vi "audio-stim2.vi"(11 "Stimulus List":dbl[][](array[numeric])=[[1.0, 3.0, 0.2, 1.0, 50.0], [2.0, 3.0, 0.2, 1.0, 100.0], [3.0, 3.0, 0.2, 1.0, 200.0], [4.0, 3.0, 0.2, 1.0, 400.0], [5.0, 3.0, 0.2, 1.0, 800.0], [6.0, 3.0, 0.2, 1.0, 1600.0], [7.0, 3.0, 0.2, 1.0, 3200.0], [8.0, 3.0, 0.2, 1.0, 6400.0], [9.0, 3.0, 0.2, 1.0, 9050.9668], [10.0, 3.0, 0.2, 1.0, 128000.0], [11.0, 3.0, 0.2, 1.0, 18101.9336], [12.0, 3.0, 0.2, 1.0, 256000.0], [13.0, 3.0, 0.2, 1.0, 36203.8672]]) -> (3 "Playing":bool=TRUE caption="Playing stimulus")   [LabVIEW 2013]
uses:
  <vilib>/DAQmx/write.llb/DAQmx Write (Digital U16 1Chan 1Samp).vi
  <vilib>/DAQmx/write.llb/DAQmx Write (Analog Wfm 1Chan NSamp).vi
  <vilib>/DAQmx/create/channels.llb/DAQmx Create Channel (AO-Voltage-Basic).vi
  <vilib>/DAQmx/create/channels.llb/DAQmx Create Channel (DO-Digital Output).vi
  <vilib>/DAQmx/miscellaneous.llb/DAQmx Fill In Error Info.vi
  <vilib>/DAQmx/configure/timing.llb/DAQmx Timing (Use Waveform).vi
panel:
  in  "Total Trials":i32=2147483647 min=1 step=1
  out "Total Played":i32 caption="Total Played or Cued"
  in  "Save Stimulus List":bool
  in  "Load Stimulus List":bool
  out "Stimulus List Path":path
  out "Log File Path":path
  in  "Play Interval Jitter (s)":dbl=0.5
  in  "Play Interval (s)":dbl=1.0
  out "error out":errorcluster
  in  "DO Ports":tag="Dev1/port0" caption="DO Ports\n(\"browse\" and select two 8 bit ports)"
  in  "Sound AO Channel":tag="Dev1/ao0"
  out "Curr Param":dbl[](array[numeric]) caption="Current (or Cued) Trial Parameters"
  in  "Sampling Rate":dbl=100000.0
  in  "stop":bool
  in  "Play":bool
  out "Current (or Cued) Waveform":waveform(dbl)(graph)={"t0"=timestamp(0 s since 1904-01-01), "dt"=1e-05, "Y"=array[19999 elements]}
  out "Waiting":bool=TRUE
  # "Stim#, Stim Type, Duration, Amplitude, Param 1, Param 2, Param 3, Param 4"
  # "Stim Type 1 DC (no parameters, just amplitude)"
  # "Stim Type 3 Pure Tone (param1 = frequency)"
  # "Stim Type 4 FM Sweep (param1 = start frequency, param2 = end frequency)"
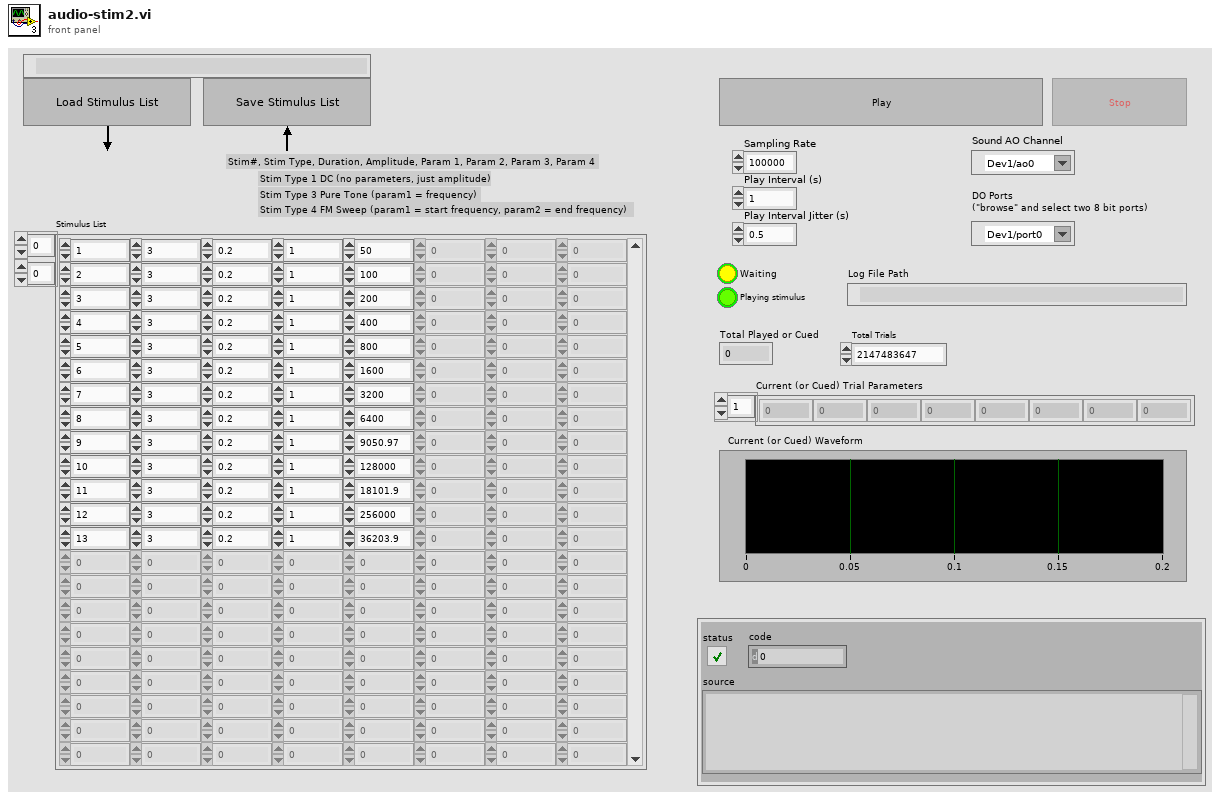
[diagram p1: front panel]
types:
  T1 = enum8{"Enabled", "Disabled", "Disabled and Grayed Out"}
  T2 = cluster{"Sampling Rate":dbl, "Value 3":dbl, dbl, "Value 2":dbl}
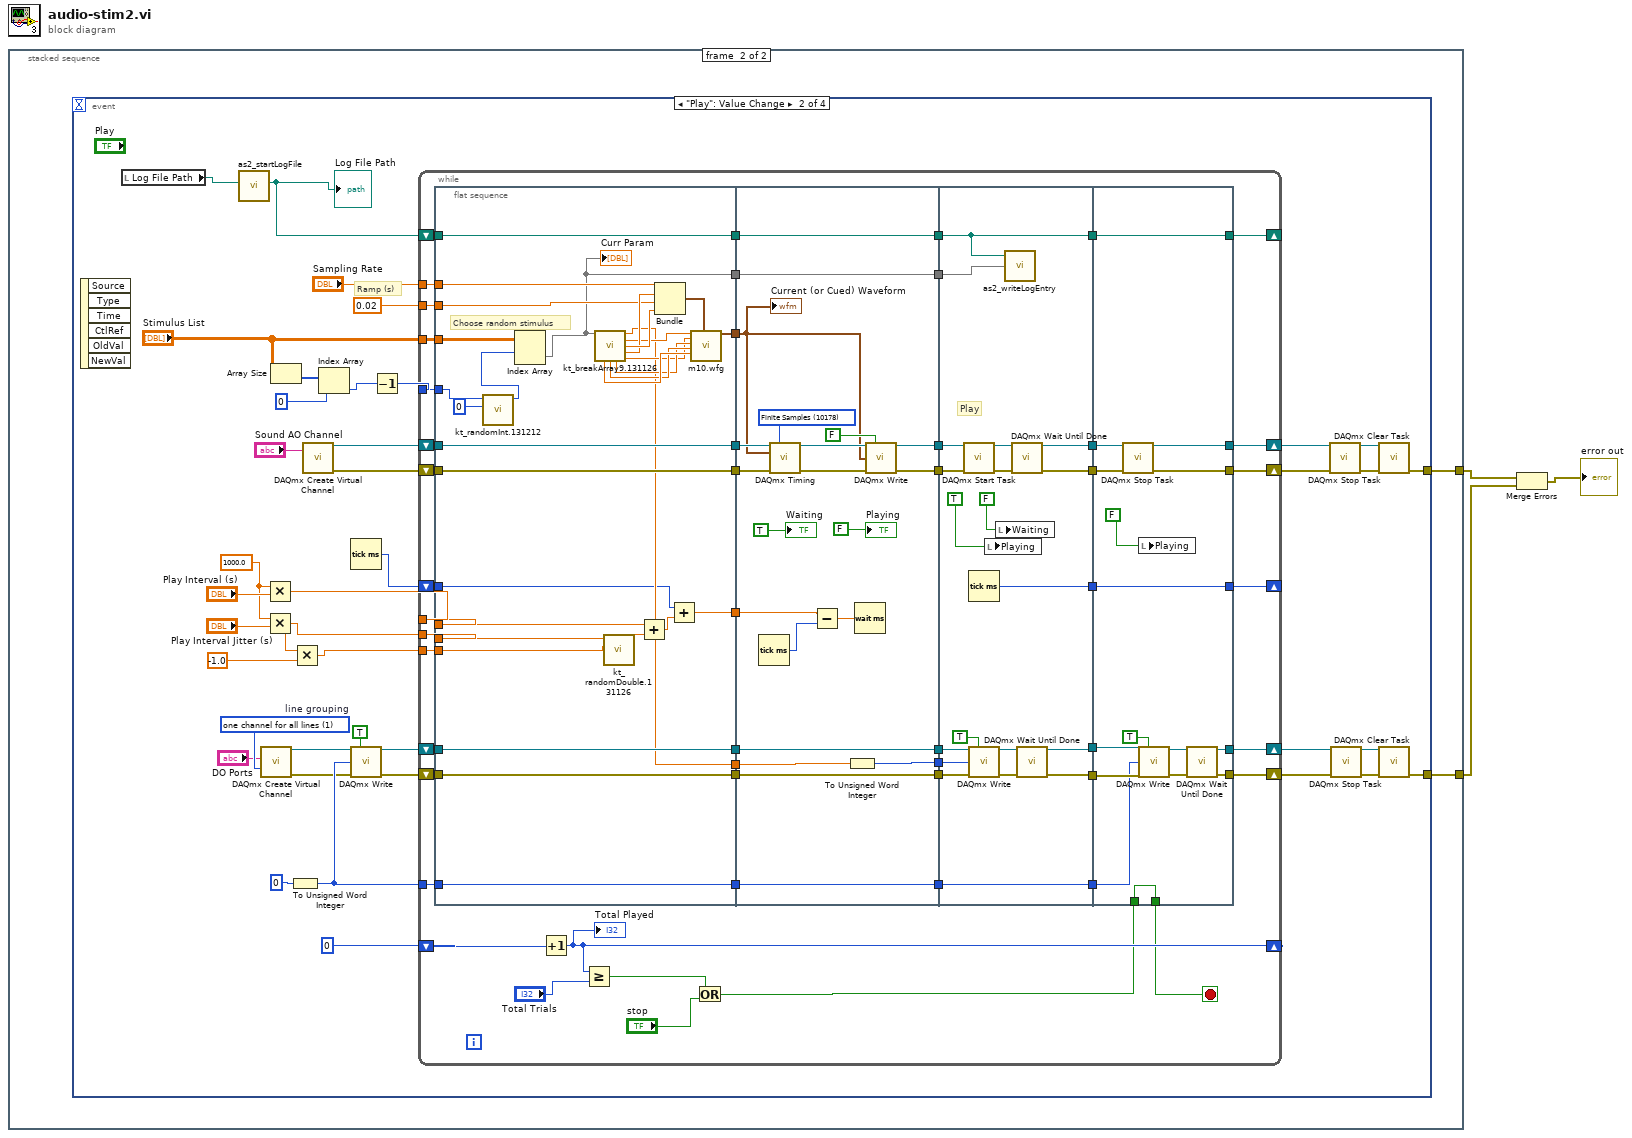
[diagram p0: block diagram]
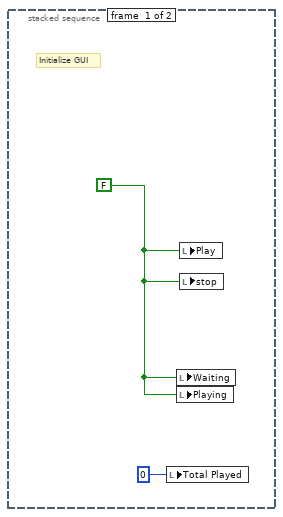
[diagram p2: hidden frame]
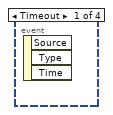
[diagram p3: hidden frame]
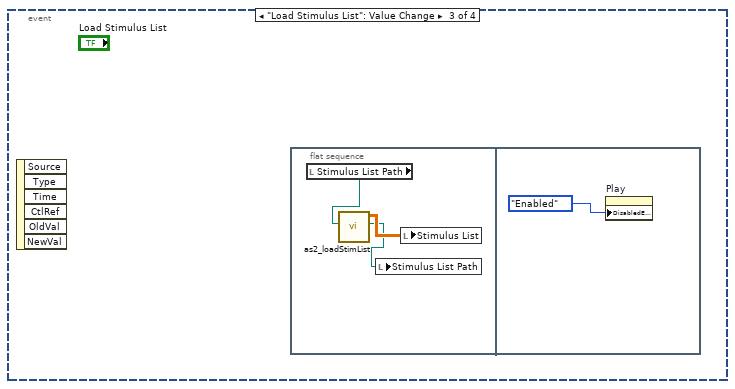
[diagram p4: hidden frame]
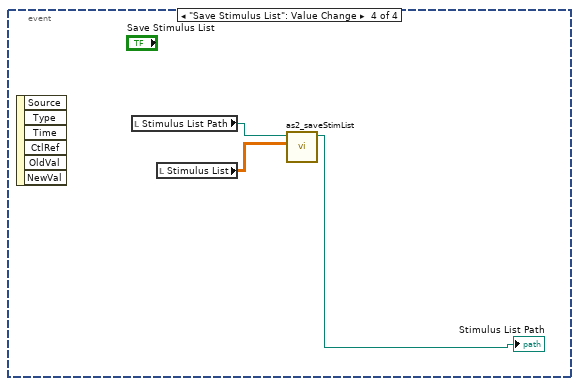
[diagram p5: hidden frame]
diagram:
  n1 = stacked-sequence {
    tunnel: [_ w7] -> w3
    tunnel: [_ w6] -> w2
    frame #0 {
      w5 = FALSE ("Play")
      # "Initialize GUI"
      n2 = local write "Total Played"(0 ("Total Played")) -> ()
      n3 = local write "Waiting"(w5) -> ()
      n4 = local write "Playing"(w5) -> ()
      n5 = local write "Play"(w5) -> ()
      n6 = local write "stop"(w5) -> ()
    }
    frame #1 {
      n7 = event shown="[1] \"Play\": Value Change" {
        selector: _ -> [_ _ _ _]
        dyn-events: _ -> [_ _ _ _]
        timeout: _ -> [_ _ _ _]
        tunnel: [_ w24 _ _] -> w7
        tunnel: [_ w23 _ _] -> w6
        event Timeout {
          n8 = event-data() -> ()  [unwired: 1 in, 3 out]
        }
        event "Play": Value Change {
          w17 = 1000.0 ("y")
          w44 = 1 items=["one channel for each line", "one channel for all lines"]  # line grouping
          # "Ramp (s)"
          n9 = event-data() -> ()  [unwired: 1 in, 6 out]
          n10 = local read "Log File Path"() -> (w12:path)
          n11 = call "as2_startLogFile.vi"("Path In"=w12) -> ("Path"=w11:path)  [unwired: 5 in, 1 out]
          "Log File Path" <- w11
          n12 = call-poly <vilib>:"DAQmx Create Virtual Channel.vi"("lines"="DO Ports", "line grouping"=w44) -> ("task out"=w22:refnum<k21>, "error out"=w21:errorcluster)  [unwired: 12 in]
          n13 = Multiply(x=w17, y="Play Interval (s)") -> (x*y=w16:dbl)
          n14 = Multiply(x=w17, y="Play Interval Jitter (s)") -> (x*y=w14:dbl)
          n15 = Array Size(array="Stimulus List") -> (size(s)=w42:i32[])
          n16 = To Unsigned Word Integer(number=u16 0 ("data")) -> (unsigned 16bit integer=w27:u16)
          n17 = Multiply(x=w14, y=-1.0) -> (x*y=w15:dbl)
          n18 = call-poly <vilib>:"DAQmx Create Virtual Channel.vi"("physical channels"="Sound AO Channel") -> ("task out"=w26:refnum<k21>, "error out"=w25:errorcluster)  [unwired: 13 in]
          n19 = Index Array(array=w42, index=0) -> (element=w10:i32)
          n20 = Tick Count (ms)() -> (millisecond timer value=w13:u32)
          n21 = call-poly <vilib>:"DAQmx Write.vi"("task/channels in"=w22, "auto start"=TRUE, "data"=w27, "error in"=w21) -> ("task out"=w31:refnum<k21>, "error out"=w30:errorcluster)  [unwired: 9 in, 1 out]
          n22 = Decrement(x=w10) -> (x-1=w9:i32)
          n23 = while {
            tunnel: "Stimulus List" -> [w72]
            tunnel: "Sampling Rate" -> [w71]
            tunnel: 0.02 -> [w70]
            shift-right: [w97] -> w36
            shift-left: w26 -> [w95]
            shift-right: [w96] -> w35
            shift-left: w25 -> [w94]
            shift-right: [w86] -> w40
            shift-left: w31 -> [w93]
            shift-right: [w85] -> w39
            shift-left: w30 -> [w80]
            shift-right: [w51] -> _
            shift-left: 0 ("data") -> [w52]
            tunnel: w27 -> [w83]
            shift-right: [w67] -> _
            shift-left: w13 -> [w66]
            tunnel: w16 -> [w62]
            tunnel: w15 -> [w63]
            tunnel: w14 -> [w64]
            shift-right: [w55] -> _
            shift-left: w11 -> [w61]
            tunnel: w9 -> [w54]
            stop <- w49 stop-if-true
            n24 = flat-sequence {
              tunnel: [w129] -> w78
              tunnel: [w128] -> w77
              tunnel: [w127] -> w76
              tunnel: [w126] -> w75
              tunnel: [w125] -> w74
              tunnel: [w117] -> w73
              tunnel: [w114] -> w69
              tunnel: [w111] -> w65
              tunnel: [w105] -> w60
              tunnel: [w104] -> w59
              tunnel: w54 -> [w103]
              tunnel: w61 -> [w105]
              tunnel: w62 -> [w106]
              tunnel: w63 -> [w109]
              tunnel: w64 -> [w110]
              tunnel: w66 -> [w112]
              tunnel: w70 -> [w115]
              tunnel: w71 -> [w116]
              tunnel: w72 -> [w101]
              tunnel: w80 -> [w125]
              tunnel: w83 -> [w126]
              tunnel: w93 -> [w127]
              tunnel: w94 -> [w128]
              tunnel: w95 -> [w129]
              tunnel: [w140] -> w99
              tunnel: [w139] -> w98
              tunnel: [w149] -> w92
              tunnel: [w148] -> w87
              tunnel: [w147] -> w84
              tunnel: [w137] -> w79
              tunnel: w78 -> [w146]
              tunnel: w77 -> [w145]
              tunnel: w76 -> [w149]
              tunnel: w75 -> [w147]
              tunnel: w74 -> [w137]
              tunnel: w73 -> [w136]
              tunnel: w69 -> [w135]
              tunnel: w65 -> [w132]
              tunnel: w60 -> [w130]
              tunnel: w59 -> [w131]
              tunnel: [w131] -> w58
              tunnel: [w130] -> w57
              tunnel: w99 -> [w160]
              tunnel: w98 -> [w159]
              tunnel: w92 -> [w168]
              tunnel: [w162] -> w91
              tunnel: [w161] -> w90
              tunnel: [w165] -> w89
              tunnel: [w164] -> w88
              tunnel: w87 -> [w169]
              tunnel: w84 -> [w163]
              tunnel: [w163] -> w82
              tunnel: w79 -> [w154]
              tunnel: [w153] -> w68
              tunnel: w58 -> [w152]
              tunnel: w57 -> [w151]
              tunnel: [w151] -> w56
              tunnel: [w174] -> w96
              tunnel: [w175] -> w97
              tunnel: w91 -> [w177]
              tunnel: w90 -> [w176]
              tunnel: w89 -> [w185]
              tunnel: w88 -> [w184]
              tunnel: [w180] -> w86
              tunnel: [w179] -> w85
              tunnel: w82 -> [w178]
              tunnel: w68 -> [w173]
              tunnel: [w173] -> w67
              tunnel: w56 -> [w172]
              tunnel: [w172] -> w55
              tunnel: w50 -> [w171]
              tunnel: [w171] -> w49
              frame #0 {
                # "Choose random stimulus"
                n25 = call "kt_randomInt.131212.vi"("Min"=0, "Max"=w103) -> ("Random"=w100:i32)  [unwired: 9 in]
                n26 = Index Array(array=w101, index (row)=w100) -> (element=w104:dbl[])  [unwired: 1 in]
                "Curr Param" <- w104
                n27 = call "kt_breakArray9.131126.vi"("Current (or Cued Trial Parameters)"=w104) -> ("Value 0"=w114:dbl, "Value 1"=w118:dbl, "Value 2"=w120:dbl, "Value 3"=w119:dbl, "Value 7"=w124:dbl, "Value 6"=w123:dbl, "Value 5"=w122:dbl, "Value 4"=w121:dbl)  [unwired: 6 in, 1 out]
                n28 = call "kt_randomDouble.131126.vi"("Min"=w109, "Max"=w110) -> ("Random"=w107:dbl)  [unwired: 9 in]
                n29 = Add(x=w106, y=w107) -> (x+y=w108:dbl)
                n30 = Bundle("Sampling Rate"=w116, "Value 3"=w119, w115, "Value 2"=w120) -> (w113:T2)  [unwired: 1 in]
                n31 = Add(x=w112, y=w108) -> (x+y=w111:dbl)
                n32 = call "m10.wfg.vi"("Stimulus Type"=w118, "Param 0"=w121, "Param 1"=w122, "Param 2"=w123, "Param 3"=w124, "Waveform Properties"=w113) -> ("Waveform Out"=w117:waveform(dbl))  [unwired: 12 in, 1 out]
              }
              frame #1 {
                w144 = 10178 items=["Finite Samples"=10178, "Continuous Samples"=10123, "Hardware Timed Single Point"=12522] ("sample mode")
                n33 = Tick Count (ms)() -> (millisecond timer value=w133:u32)
                n34 = call-poly <vilib>:"DAQmx Timing.vi"("task/channels in"=w146, "sample mode"=w144, "waveform"=w136, "error in"=w145) -> ("task out"=w143:refnum<k21>, "error out"=w142:errorcluster)  [unwired: 10 in]
                n35 = Subtract(x=w132, y=w133) -> (x-y=w134:dbl)
                n36 = To Unsigned Word Integer(number=w135) -> (unsigned 16bit integer=w148:u16)
                n37 = Wait (ms)(milliseconds to wait=w134) -> ()  [unwired: 1 out]
                n38 = call-poly <vilib>:"DAQmx Write.vi"("task/channels in"=w143, "auto start"=FALSE, "data"=w136, "error in"=w142) -> ("task out"=w140:refnum<k21>, "error out"=w139:errorcluster)  [unwired: 9 in, 1 out]
                "Waiting" <- TRUE ("Playing Stimulus")
                "Playing" <- FALSE ("Playing Stimulus")
                "Current (or Cued) Waveform" <- w136
              }
              frame #2 {
                # "Play"
                n39 = call <vilib>:"DAQmx Start Task.vi"("task/channels in"=w160, "error in"=w159) -> ("task out"=w158:refnum<k21>, "error out"=w157:errorcluster)  [unwired: 12 in]
                n40 = Tick Count (ms)() -> (millisecond timer value=w153:u32)
                n41 = call-poly <vilib>:"DAQmx Write.vi"("task/channels in"=w168, "auto start"=TRUE, "data"=w169, "error in"=w154) -> ("task out"=w167:refnum<k21>, "error out"=w166:errorcluster)  [unwired: 9 in, 1 out]
                n42 = local write "Playing"(TRUE ("Playing Stimulus")) -> ()
                n43 = local write "Waiting"(FALSE ("Playing Stimulus")) -> ()
                n44 = call "as2_writeLogEntry.vi"("Path In"=w151, "Curr Param"=w152) -> ()  [unwired: 4 in, 1 out]
                n45 = call <vilib>:"DAQmx Wait Until Done.vi"("task/channels in"=w158, "error in"=w157) -> ("task out"=w162:refnum<k21>, "error out"=w161:errorcluster)  [unwired: 12 in]
                n46 = call <vilib>:"DAQmx Wait Until Done.vi"("task/channels in"=w167, "error in"=w166) -> ("task out"=w165:refnum<k21>, "error out"=w164:errorcluster)  [unwired: 12 in]
              }
              frame #3 {
                n47 = call <vilib>:"DAQmx Stop Task.vi"("task/channels in"=w177, "error in"=w176) -> ("task out"=w175:refnum<k21>, "error out"=w174:errorcluster)  [unwired: 12 in]
                n48 = local write "Playing"(FALSE ("Playing Stimulus")) -> ()
                n49 = call-poly <vilib>:"DAQmx Write.vi"("task/channels in"=w185, "auto start"=TRUE, "data"=w178, "error in"=w184) -> ("task out"=w182:refnum<k21>, "error out"=w181:errorcluster)  [unwired: 9 in, 1 out]
                n50 = call <vilib>:"DAQmx Wait Until Done.vi"("task/channels in"=w182, "error in"=w181) -> ("task out"=w180:refnum<k21>, "error out"=w179:errorcluster)  [unwired: 12 in]
              }
            }
            n51 = Increment(x=w52) -> (x+1=w51:i32)
            "Total Played" <- w51
            n52 = Greater Or Equal?(x=w51, y="Total Trials") -> (x >= y?=w81:bool)
            n53 = Or(x=w81, y="stop") -> (x .or. y?=w50:bool)
          }
          n54 = call <vilib>:"DAQmx Stop Task.vi"("task/channels in"=w36, "error in"=w35) -> ("task out"=w34:refnum<k21>, "error out"=w33:errorcluster)  [unwired: 12 in]
          n55 = call <vilib>:"DAQmx Stop Task.vi"("task/channels in"=w40, "error in"=w39) -> ("task out"=w38:refnum<k21>, "error out"=w37:errorcluster)  [unwired: 12 in]
          n56 = call <vilib>:"DAQmx Clear Task.vi"("task in"=w34, "error in"=w33) -> ("error out"=w24:errorcluster)  [unwired: 13 in]
          n57 = call <vilib>:"DAQmx Clear Task.vi"("task in"=w38, "error in"=w37) -> ("error out"=w23:errorcluster)  [unwired: 13 in]
        }
        event "Load Stimulus List": Value Change {
          n58 = event-data() -> ()  [unwired: 1 in, 6 out]
          n59 = flat-sequence {
            frame #0 {
              n60 = local read "Stimulus List Path"() -> (w189:path)
              n61 = call "as2_loadStimList.vi"("Path In"=w189) -> ("Path"=w187:path, "Stimulus List"=w188:dbl[][])  [unwired: 4 in, 1 out]
              n62 = local write "Stimulus List Path"(w187) -> ()
              n63 = local write "Stimulus List"(w188) -> ()
            }
            frame #1 {
              n64 = property on="Play" class="Bool (strict)"("DisabledEnum"=T1."Enabled" ("Disabled")) -> ()  [unwired: 2 in, 2 out]
            }
          }
        }
        event "Save Stimulus List": Value Change {
          n65 = event-data() -> ()  [unwired: 1 in, 6 out]
          n66 = local read "Stimulus List Path"() -> (w193:path)
          n67 = local read "Stimulus List"() -> (w192:dbl[][])
          n68 = call "as2_saveStimList.vi"("Stimulus List"=w192, "Path In"=w193) -> ("Path"=→"Stimulus List Path":path)  [unwired: 4 in, 1 out]
        }
      }
    }
  }
  n69 = Merge Errors(w3, w2) -> (→"error out":errorcluster)
